vi "ParseCSVNumberString.vi"(8 "error in":errorcluster, 9 "NotANumberDefault":dbl=-1.0, 10 "Expected Size":dbl=6.0, 11 "String":string) -> (0 "error out":errorcluster, 3 "Array":u16[](array[numeric]))   [LabVIEW 2018]
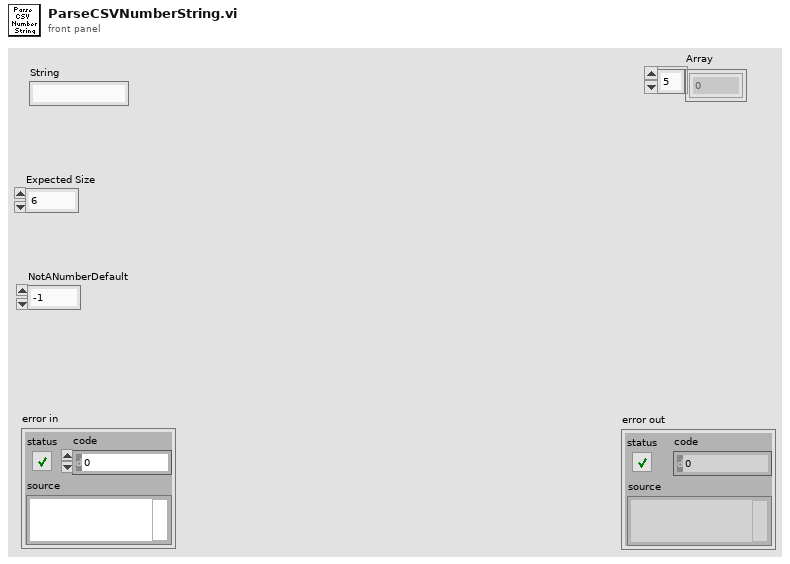
[diagram p1: front panel]
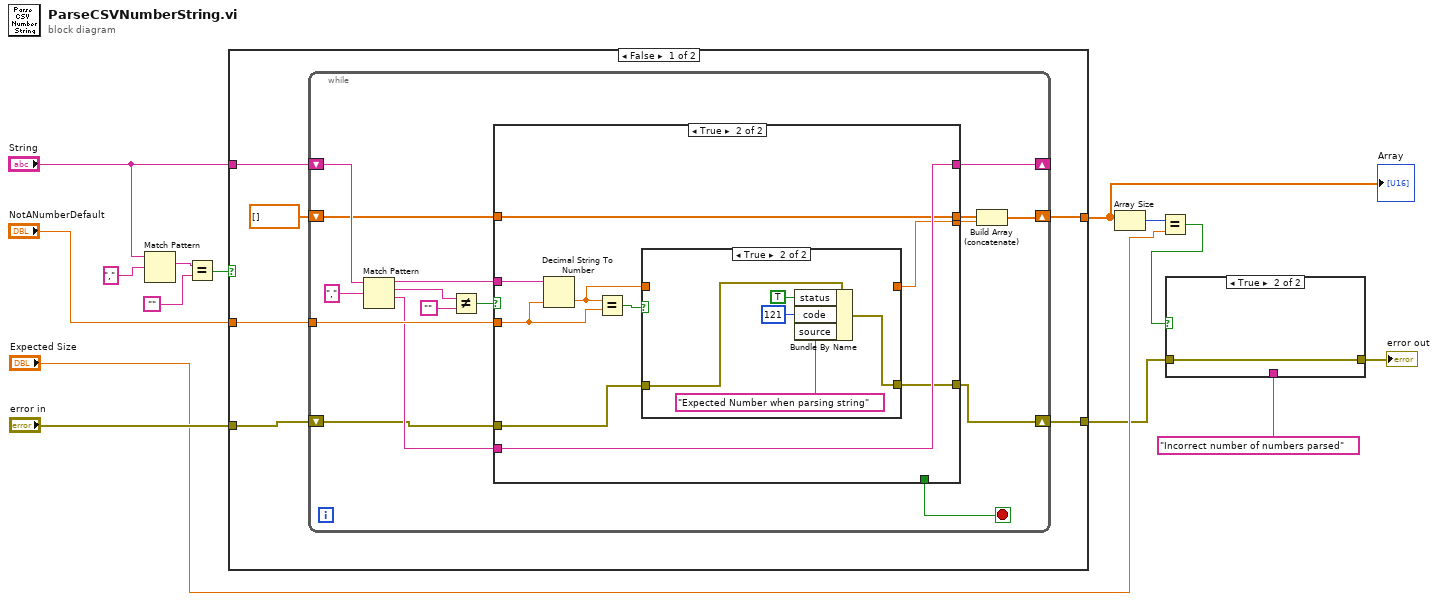
[diagram p0: block diagram]
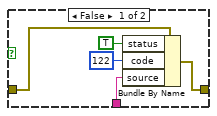
[diagram p2: hidden frame]
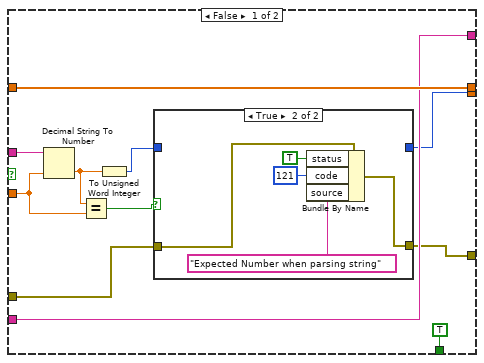
[diagram p3: hidden frame]
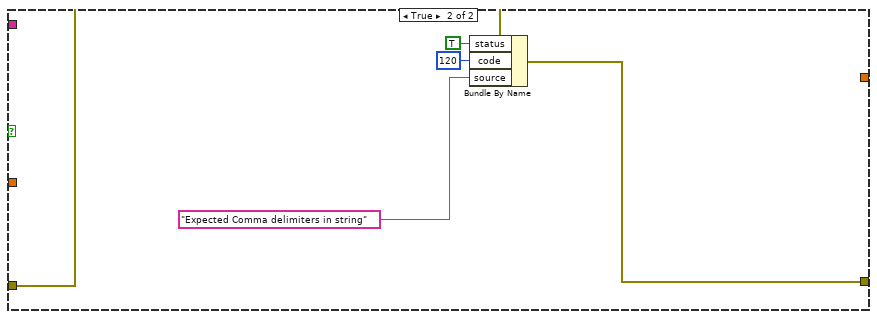
[diagram p6: hidden frame]
diagram:
  n1 = Match Pattern(string="String", regular expression=",") -> (match substring=w10:string)  [unwired: 1 in, 3 out]
  n2 = Equal?(x=w10, y="") -> (x = y?=w9:bool)
  n3 = case shown="False" w9 {
    tunnel: "NotANumberDefault" -> [w20 _]
    tunnel: "String" -> [w19 _]
    tunnel: "error in" -> [w17 w75]
    tunnel: [w16 w74] -> w3
    tunnel: [w18 _] -> w7
    frame False {
      n4 = while {
        tunnel: w20 -> [w33]
        shift-right: [w28] -> _
        shift-left: w19 -> [w34]
        shift-right: [w26] -> w18
        shift-left: dbl[] [] -> [w24]
        shift-right: [w21] -> w16
        shift-left: w17 -> [w22]
        stop <- w27 stop-if-true
        n5 = Match Pattern(string=w34, regular expression=",") -> (before substring=w35:string, match substring=w31:string, after substring=w29:string)  [unwired: 1 in, 1 out]
        n6 = Not Equal?(x=w31, y="") -> (x != y?=w32:bool)
        n7 = case shown="True" w32 {
          tunnel: w35 -> [w46 w63]
          tunnel: w33 -> [w43 w61]
          tunnel: w29 -> [w44 w62]
          tunnel: [w44 w62] -> w28
          tunnel: [TRUE _] -> w27
          tunnel: [w38 w56] -> w25
          tunnel: w24 -> [w45 w59]
          tunnel: [w45 w59] -> w23
          tunnel: w22 -> [w42 w58]
          tunnel: [w41 w57] -> w21
          frame False {
            n8 = Decimal String To Number(string=w46, default (0L)=w43) -> (number=w37:dbl)  [unwired: 1 in, 1 out]
            n9 = Equal?(x=w37, y=w43) -> (x = y?=w40:bool)
            n10 = To Unsigned Word Integer(number=w37) -> (unsigned 16bit integer=w39:u16)
            n11 = case shown="True" w40 {
              tunnel: w42 -> [w49 w54]
              tunnel: [w49 w53] -> w41
              tunnel: w39 -> [w48 _]
              tunnel: [w48 _] -> w38
              frame False {
              }
              frame True {
                n12 = Bundle By Name(cluster=w54, "status"=TRUE, "code"=121, "source"="Expected Number when parsing string") -> (w53:errorcluster)
              }
            }
          }
          frame True {
            n13 = Decimal String To Number(string=w63, default (0L)=w61) -> (number=w55:dbl)  [unwired: 1 in, 1 out]
            n14 = Equal?(x=w55, y=w61) -> (x = y?=w60:bool)
            n15 = case shown="True" w60 {
              tunnel: w58 -> [w65 w70]
              tunnel: [w65 w69] -> w57
              tunnel: w55 -> [w64 _]
              tunnel: [w64 _] -> w56
              frame False {
              }
              frame True {
                n16 = Bundle By Name(cluster=w70, "status"=TRUE, "code"=121, "source"="Expected Number when parsing string") -> (w69:errorcluster)
              }
            }
          }
        }
        n17 = Build Array (concatenate)(w23, w25) -> (w26:dbl[])
      }
    }
    frame True {
      n18 = Bundle By Name(cluster=w75, "status"=TRUE, "code"=120, "source"="Expected Comma delimiters in string") -> (w74:errorcluster)
    }
  }
  "Array" <- w7
  n19 = Array Size(array=w7) -> (size(s)=w6:i32)
  n20 = Equal?(x=w6, y="Expected Size") -> (x = y?=w4:bool)
  n21 = case shown="True" w4 {
    tunnel: w3 -> [w80 w81]
    tunnel: [w79 w81] -> w2
    tunnel: "Incorrect number of numbers parsed" ("source") -> [w76 _]
    frame False {
      n22 = Bundle By Name(cluster=w80, "status"=TRUE, "code"=122, "source"=w76) -> (w79:errorcluster)
    }
    frame True {
    }
  }
  "error out" <- w2
